vi "Output Stream Control.vi"(0 "start trigger":bool, 1 "reset":bool, 5 "burst size":u32, 7 "abort":bool, 9 "ready to read stream (T)":bool=TRUE, 11 "fifo output valid":bool, 12 "samples per cycle":u32=1) -> (4 "read stream":bool, 6 "state":T1, 8 "samples processed":u32, 10 "number of underflows":u32, 15 "fifo underflow":bool)   [LabVIEW 2023]
doc: "Controls whether data is read from the DMA FIFO for the generation stream. If the burst size is zero, a continuous generation is initiated when you set the <B>start trigger</B> parameter to TRUE. If the burst size is greater than zero, the generation occurs in bursts of the designated size, and is initiated when the internal state machine is idle and a start trigger is received.\n\nThis VI indicates whether an underflow occurred in the generation and returns the number of underflows that have occurred.\n\nThe internal state machine returns the number of samples processed since the beginning of the most recent generation and also the current state of the state machine.\n\n<B>Input Parameters</B>\n\n<B>start trigger</B> transitions the stream to an active state when asserted.\n\n<B>burst size</B> is the number of samples to generate.\n\n<B>abort</B> stops the generation.\n\n<B>ready to read stream</B> is wired to 'read stream' when the stream is active.\n\n<B>fifo output valid</B> helps count underflows. Wire to Read FIFO's 'output valid'.\n\n<B>reset</B> the stream to Idle and set counters to zero.\n\n<B>samples per cycle</B> is the number of samples to be processed per clock cycle. This value is based on how many samples your front-end generates per clock cycles and is likely a constant.\n\n<B>Output Parameters</B>\n\n<B>read stream</B> is a flow control signal to control whether data is read from the DMA FIFO.\n\n<B>state</B> of the output stream controller.\n\n<B>samples processed</B> is the number of samples processed by the Tx signal chain.\n\n<B>number of underflows</B> is the count of FIFO underflows.\n\n<B>fifo underflow</B> indicates whether there was a FIFO underflow on the last write."
uses:
  <instrlib>/niUSRP/Reference FPGA/USRPRIO Sample VIs/FPGA/SubVIs/Stream Control State.ctl
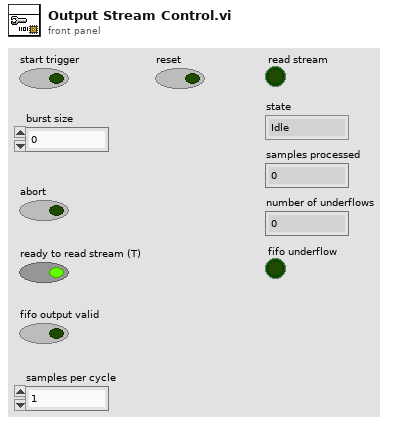
[diagram p1: front panel]
types:
  T1 = typedef "Stream Control State.ctl" = enum16{"Idle", "Active"}
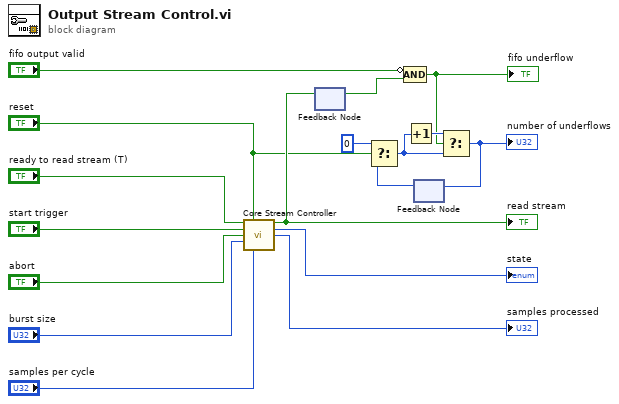
[diagram p0: block diagram]
diagram:
  n1 = call <instrlib>:"Core Stream Controller.vi"("input valid"="ready to read stream (T)", "reset"="reset", "start trigger"="start trigger", "abort"="abort", "burst size"="burst size", "samples per cycle"="samples per cycle") -> ("write stream"=w12:bool, "state"=→"state":T1, "samples processed"=→"samples processed":u32)  [unwired: 7 in]
  "read stream" <- w12
  n2 = feedback-in #1(w12) -> ()
  n3 = feedback #1() -> (w11:bool)  [unwired: 1 in]
  n4 = Compound Arithmetic op=AND(invert "fifo output valid", w11) -> (w4:bool)
  "fifo underflow" <- w4
  n5 = feedback #2() -> (w7:u32)  [unwired: 1 in]
  n6 = Select(t=u32 0, s="reset", f=w7) -> (s? t:f=w6:u32)
  n7 = Increment(x=w6) -> (x+1=w9:u32)
  n8 = Select(t=w9, s=w4, f=w6) -> (s? t:f=w8:u32)
  "number of underflows" <- w8
  n9 = feedback-in #2(w8) -> ()
